vi "VMC-5.vi"(11 "数组":u8[](array[numeric])) -> (1 "对准数据来源字":cluster{"位置数据":string, "姿态数据":string}, 2 "系统状态":cluster{"工作状态":string, "工作模式":string}, 3 "字符串":string, 4 "组合数据来源":T1)   [LabVIEW 2012]
uses:
  index-i16.vi
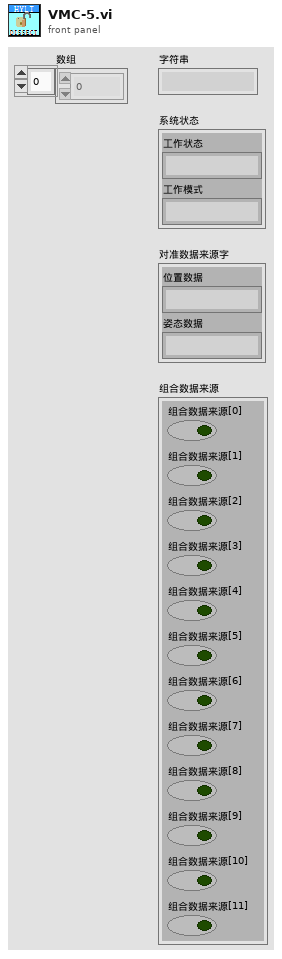
[diagram p1: front panel]
types:
  T1 = cluster{"组合数据来源[0]":bool, "组合数据来源[1]":bool, "组合数据来源[2]":bool, "组合数据来源[3]":bool, "组合数据来源[4]":bool, "组合数据来源[5]":bool, "组合数据来源[6]":bool, "组合数据来源[7]":bool, "组合数据来源[8]":bool, "组合数据来源[9]":bool, "组合数据来源[10]":bool, "组合数据来源[11]":bool}
  T2 = cluster{"GNSS1+GPS":bool, "GNSS1BD":bool, "GCSS1+GLO":bool, "GNSS3+GPS":bool, "GNSS2+GPS":bool, "GNSS2BD":bool, "GNSS2+GLO":bool, "GNSS3BD":bool, "GNSS3+GLO":bool, "大气数据":bool, "星敏1数据":bool, "星敏2数据":bool}
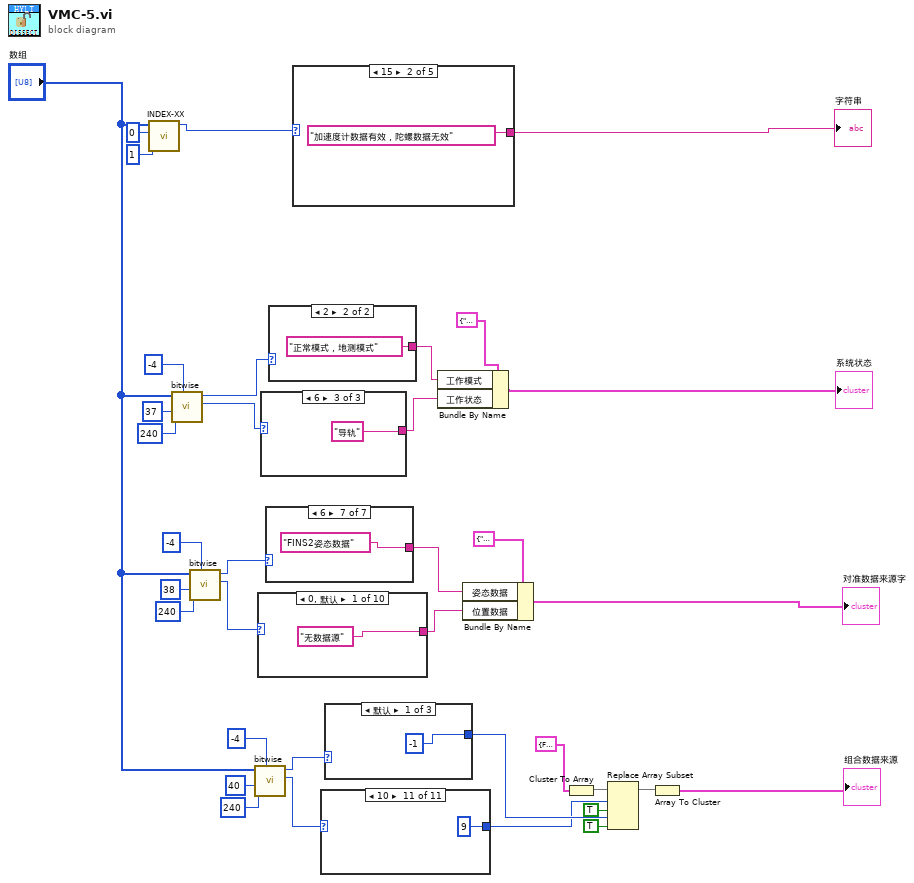
[diagram p0: block diagram]
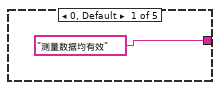
[diagram p2: hidden frame]
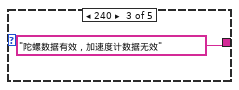
[diagram p3: hidden frame]
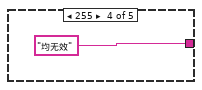
[diagram p4: hidden frame]
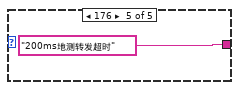
[diagram p5: hidden frame]
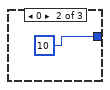
[diagram p6: hidden frame]
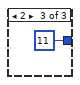
[diagram p7: hidden frame]
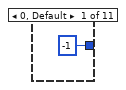
[diagram p8: hidden frame]
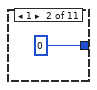
[diagram p9: hidden frame]
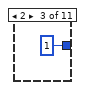
[diagram p10: hidden frame]
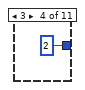
[diagram p11: hidden frame]
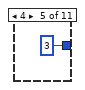
[diagram p12: hidden frame]
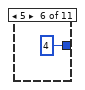
[diagram p13: hidden frame]
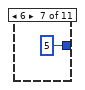
[diagram p14: hidden frame]
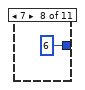
[diagram p15: hidden frame]
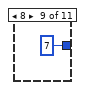
[diagram p16: hidden frame]
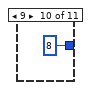
[diagram p17: hidden frame]
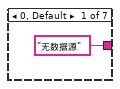
[diagram p18: hidden frame]
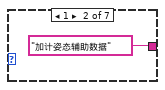
[diagram p19: hidden frame]
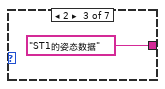
[diagram p20: hidden frame]
diagram:
  n1 = call-poly "INDEX-XX.vi"("长度"=1, "索引"=0, "数组"="数组") -> ("数值输出"=w36:i16)  [unwired: 8 in]
  n2 = call "bitwise.vi"("移位"=i16 -4, "置1"=u8 240, "索引"=37, "数组"="数组") -> ("y2"=w2:u8, "y1"=w3:u8)  [unwired: 6 in]
  n3 = call "bitwise.vi"("移位"=i16 -4, "置1"=u8 240, "索引"=38, "数组"="数组") -> ("y2"=w25:u8, "y1"=w24:u8)  [unwired: 6 in]
  n4 = call "bitwise.vi"("移位"=i16 -4, "置1"=u8 240, "索引"=40, "数组"="数组") -> ("y2"=w27:u8, "y1"=w26:u8)  [unwired: 6 in]
  n5 = case shown="0, 默认" w25 {
    tunnel: ["无数据源" "GNSS1的GPS数据" "GNSS2的GPS数据" "GNSS3的GPS数据" "GNSS1的BD数据" "GNSS2的BD数据" "GNSS3的BD数据" "GNSS1的GLONASS数据" "GNSS2的GLONASS数据" "GNSS3的GLONASS数据"] -> w7
    frame 0, Default {
    }
    frame 1 {
    }
    frame 2 {
    }
    frame 3 {
    }
    frame 4 {
    }
    frame 5 {
    }
    frame 6 {
    }
    frame 7 {
    }
    frame 8 {
    }
    frame 9 {
    }
  }
  n6 = case shown="6" w2 {
    tunnel: ["N/A,准备" "罗经对准，在轨对准" "导轨"] -> w4
    frame 4, Default {
    }
    frame 5 {
    }
    frame 6 {
    }
  }
  n7 = case shown="6" w24 {
    tunnel: ["无数据源" "加计姿态辅助数据" "ST1的姿态数据" "ST2的姿态数据" "LINS姿态数据" "FINS1姿态数据" "FINS2姿态数据"] -> w8
    frame 0, Default {
    }
    frame 1 {
    }
    frame 2 {
    }
    frame 3 {
    }
    frame 4 {
    }
    frame 5 {
    }
    frame 6 {
    }
  }
  n8 = case shown="2" w3 {
    tunnel: ["未知" "正常模式，地测模式"] -> w5
    frame 0, Default {
    }
    frame 2 {
    }
  }
  n9 = case shown="15" w36 {
    tunnel: ["测量数据均有效" "加速度计数据有效，陀螺数据无效" "陀螺数据有效，加速度计数据无效" "均无效" "200ms地测转发超时"] -> w1
    frame 0, Default {
    }
    frame 15 {
    }
    frame 240 {
    }
    frame 255 {
    }
    frame 176 {
    }
  }
  "字符串" <- w1
  n10 = case shown="10" w27 {
    tunnel: [-1 0 1 2 3 4 5 6 7 8 9] -> w11
    frame 0, Default {
    }
    frame 1 {
    }
    frame 2 {
    }
    frame 3 {
    }
    frame 4 {
    }
    frame 5 {
    }
    frame 6 {
    }
    frame 7 {
    }
    frame 8 {
    }
    frame 9 {
    }
    frame 10 {
    }
  }
  n11 = case shown="默认" w26 {
    tunnel: [-1 10 11] -> w14
    frame Default {
    }
    frame 0 {
    }
    frame 2 {
    }
  }
  n12 = Bundle By Name(cluster=cluster{"工作状态":string, "工作模式":string} {"工作状态"="", "工作模式"=""} ("系统状态"), "工作模式"=w5, "工作状态"=w4) -> (→"系统状态":cluster{"工作状态":string, "工作模式":string})
  n13 = Bundle By Name(cluster=cluster{"位置数据":string, "姿态数据":string} {"位置数据"="", "姿态数据"=""} ("数据来源"), "姿态数据"=w8, "位置数据"=w7) -> (→"对准数据来源字":cluster{"位置数据":string, "姿态数据":string})
  n14 = Cluster To Array(cluster=T2 {"GNSS1+GPS"=FALSE, "GNSS1BD"=FALSE, "GCSS1+GLO"=FALSE, "GNSS3+GPS"=FALSE, "GNSS2+GPS"=FALSE, "GNSS2BD"=FALSE, "GNSS2+GLO"=FALSE, "GNSS3BD"=FALSE, "GNSS3+GLO"=FALSE, "大气数据"=FALSE, "星敏1数据"=FALSE, "星敏2数据"=FALSE} ("组合数据来源")) -> (array=w9:bool[])
  n15 = Replace Array Subset(array=w9, new element #1=TRUE ("新元素/子数组"), index #1=w11, new element #2=TRUE ("新元素/子数组"), index #2=w14) -> (w12:bool[])
  n16 = Array To Cluster(array=w12) -> (cluster=→"组合数据来源":T1)
